vi "XY Graph Get Plot(s) from Headerless String Array.vi"(4 "Default X step (1)":dbl=1.0, 6 "Default X start (0)":dbl, 7 "Alternating Axes?":bool, 8 "error in (no error)":errorcluster, 9 "Delimiter":string, 10 "Abscissa Column? (T)":bool=TRUE, 11 "Text Lines":string[](array[string])) -> (0 "error out":errorcluster, 3 "Plot Array":cluster{"Array":dbl[], "Array":dbl[]}[](array[cluster]))   [LabVIEW 2021, in "XY Graph Add-Ons.lvlib"]
uses:
  XY Graph Add-Ons.lvlib
  1475674b-5358-4f42-8095-6f5b9cc962ed.vi
  95ffc780-ba50-4d26-8739-638f745671cb.vi
  <vilib>/Utility/error.llb/Error Cluster From Error Code.vi
  <vilib>/ErrorRing/Error Ring.xnode
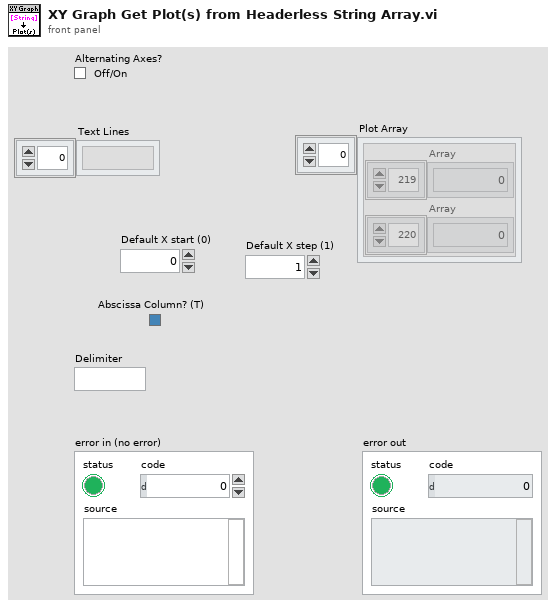
[diagram p1: front panel]
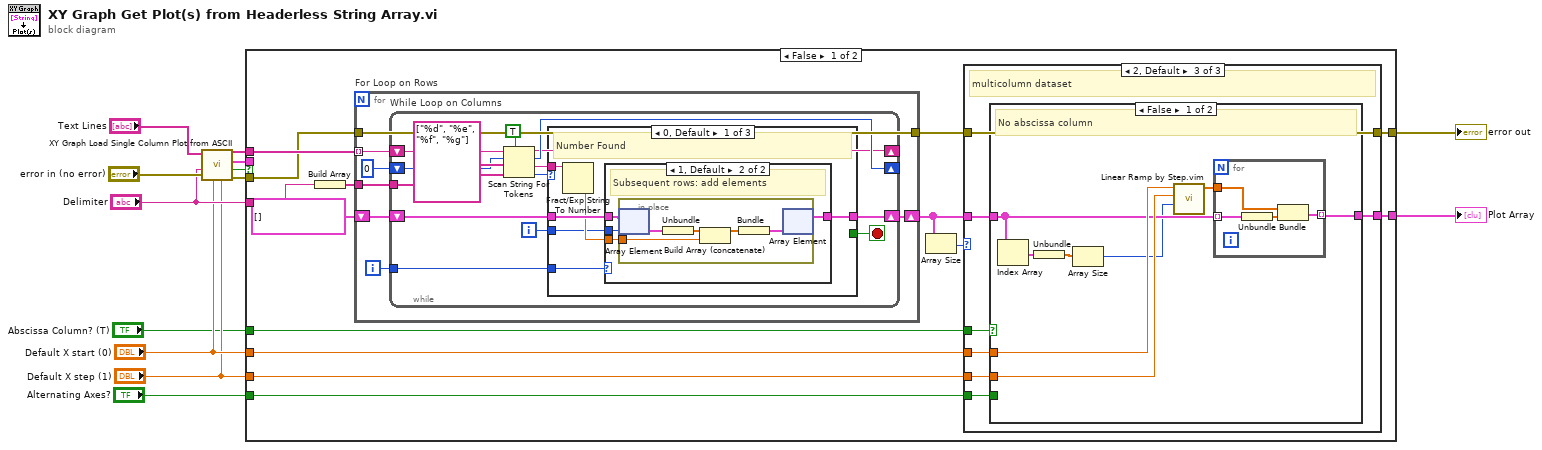
[diagram p0: block diagram]
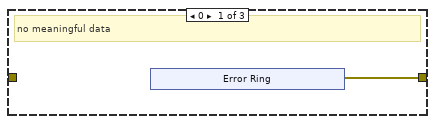
[diagram p2: hidden frame]
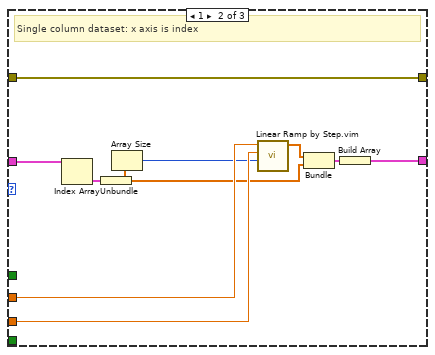
[diagram p3: hidden frame]
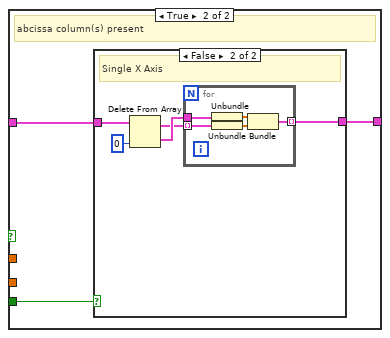
[diagram p4: hidden frame]
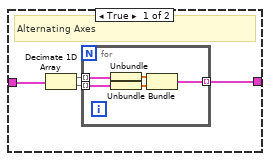
[diagram p5: hidden frame]
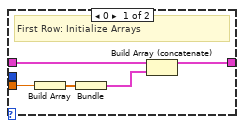
[diagram p6: hidden frame]
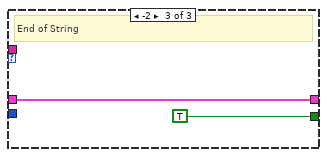
[diagram p8: hidden frame]
diagram:
  n1 = call "XY Graph Load Single Column Plot from ASCII.vi"("Default X step (1)"="Default X step (1)", "Default X start (0)"="Default X start (0)", "error in (no error)"="error in (no error)", "Delimiter (TAB)"="Delimiter", "String Array"="Text Lines") -> ("error out"=w8:errorcluster, "Single Column?"=w9:bool, "Plot Array"=w10:cluster{"Array":dbl[], "Array":dbl[]}[], "String Array dup"=w13:string[])  [unwired: 3 in]
  n2 = case shown="False" w9 {
    tunnel: [w27 w129] -> w4
    tunnel: "Alternating Axes?" -> [w26 _]
    tunnel: [w25 w128] -> w6
    tunnel: w13 -> [w19 _]
    tunnel: "Delimiter" -> [w18 _]
    tunnel: w8 -> [w17 w128]
    tunnel: w10 -> [_ w129]
    tunnel: "Default X start (0)" -> [w16 _]
    tunnel: "Default X step (1)" -> [w15 _]
    tunnel: "Abscissa Column? (T)" -> [w14 _]
    frame False {
      n3 = Build Array(w18) -> (w24:string[])
      n4 = for "For Loop on Rows" {
        tunnel: w19 -> [w90] mode=indexing
        tunnel: w24 -> [w89]
        shift-right: [w86] -> w22
        shift-left: cluster{dbl[]}[] [] -> [w87]
        tunnel: w17 -> [w84]
        tunnel: [w84] -> w20
        i -> [w85]
        n5 = while "While Loop on Columns" {
          tunnel: w89 -> [w103]
          shift-right: [w99] -> _
          shift-left: w90 -> [w104]
          shift-right: [w100] -> _
          shift-left: 0 ("offset past token") -> [w101]
          shift-right: [w93] -> w86
          shift-left: w87 -> [w95]
          tunnel: w85 -> [w92]
          i -> [w94]
          stop <- w96 stop-if-true
          n6 = Scan String For Tokens(5:TRUE ("allow empty tokens? (F)"), 6:w103, 7:string[] ["%d", "%e", "%f", "%g"] ("operators (none)"), 8:w101, 9:w104) -> (0:w98:i32, 1:w97:string, 2:w100:i32, 3:w99:string)  [unwired: 1 in]
          n7 = case shown="0, Default" w98 {
            tunnel: w97 -> [w110 _ _]
            tunnel: [_ _ TRUE] -> w96
            tunnel: w95 -> [w109 w125 w126]
            tunnel: w94 -> [w106 _ _]
            tunnel: [w107 w125 w126] -> w93
            tunnel: w92 -> [w105 _ _]
            frame 0, Default {
              # "Number Found"
              n8 = Fract/Exp String To Number(string=w110) -> (number=w108:dbl)  [unwired: 3 in, 1 out]
              n9 = case shown="1, Default" w105 {
                tunnel: w109 -> [w113 w119]
                tunnel: w108 -> [w115 w118]
                tunnel: [w111 w117] -> w107
                tunnel: w106 -> [_ w116]
                frame 0 {
                  # "First Row: Initialize Arrays"
                  n10 = Build Array(w115) -> (w114:dbl[])
                  n11 = Bundle(w114) -> (w112:cluster{dbl[]})  [unwired: 1 in]
                  n12 = Build Array (concatenate)(w113, w112) -> (w111:cluster{dbl[]}[])
                }
                frame 1, Default {
                  # "Subsequent rows: add elements"
                  n13 = in-place {
                    in-place-border: w118 -> [w123]
                    n14 = in-place-array #1(w119, w116) -> (w124:cluster{dbl[]})
                    n15 = Unbundle(w124) -> (w121:dbl[])
                    n16 = Build Array (concatenate)(w121, w123) -> (w122:dbl[])
                    n17 = Bundle(w122) -> (w120:cluster{dbl[]})  [unwired: 1 in]
                    n18 = in-place-array #1(w120) -> (w117:cluster{dbl[]}[])  [unwired: 1 out]
                  }
                }
              }
            }
            frame -1 {
              # "Some columns have less numbers than others"
              # "Number not Found"
            }
            frame -2 {
              # "End of String"
            }
          }
        }
      }
      n19 = Array Size(array=w22) -> (size(s)=w21:i32)
      n20 = case shown="2, Default" w21 {
        tunnel: [_ w39 w49] -> w27
        tunnel: w26 -> [_ _ w48]
        tunnel: w22 -> [_ w42 w47]
        tunnel: w20 -> [_ w38 w46]
        tunnel: [w28 w38 w46] -> w25
        tunnel: w16 -> [_ w37 w44]
        tunnel: w15 -> [_ w36 w43]
        tunnel: w14 -> [_ _ w45]
        frame 0 {
          # "no meaningful data"
          n21 = xnode "Error Ring"() -> ("error out"=w28:errorcluster)
        }
        frame 1 {
          # "Single column dataset: x axis is index"
          n22 = Index Array(array=w42) -> (element=w41:cluster{dbl[]})  [unwired: 1 in]
          n23 = Unbundle(w41) -> (w35:dbl[])
          n24 = Array Size(array=w35) -> (size(s)=w34:i32)
          n25 = call "Linear Ramp by Step.vim"("# Elements (1)"=w34, "Step (1)"=w36, "Start (0)"=w37) -> ("Ramp"=w33:dbl[])  [unwired: 8 in]
          n26 = Bundle("Ramp"=w33, w35) -> (w40:cluster{"Ramp":dbl[], dbl[]})  [unwired: 1 in]
          n27 = Build Array(w40) -> (w39:cluster{"Ramp":dbl[], dbl[]}[])
        }
        frame 2, Default {
          # "multicolumn dataset"
          n28 = case shown="False" w45 {
            tunnel: [w50 w64] -> w49
            tunnel: w48 -> [_ w63]
            tunnel: w47 -> [w55 w62]
            tunnel: w44 -> [w57 _]
            tunnel: w43 -> [w56 _]
            frame False {
              # "No abscissa column"
              n29 = Index Array(array=w55) -> (element=w54:cluster{dbl[]})  [unwired: 1 in]
              n30 = Unbundle(w54) -> (w53:dbl[])
              n31 = Array Size(array=w53) -> (size(s)=w52:i32)
              n32 = call "Linear Ramp by Step.vim"("# Elements (1)"=w52, "Step (1)"=w56, "Start (0)"=w57) -> ("Ramp"=w51:dbl[])  [unwired: 8 in]
              n33 = for {
                tunnel: w55 -> [w61] mode=indexing
                tunnel: [w59] -> w50 mode=indexing
                tunnel: w51 -> [w58]
                n34 = Unbundle(w61) -> (w60:dbl[])
                n35 = Bundle("Ramp"=w58, w60) -> (w59:cluster{"Ramp":dbl[], dbl[]})  [unwired: 1 in]
              }
            }
            frame True {
              # "abcissa column(s) present"
              n36 = case shown="False" w63 {
                tunnel: w62 -> [w68 w77]
                tunnel: [w65 w78] -> w64
                frame True {
                  # "Alternating Axes"
                  n37 = Decimate 1D Array(w68) -> (w67:cluster{dbl[]}[], w66:cluster{dbl[]}[])
                  n38 = for {
                    tunnel: w67 -> [w73] mode=indexing
                    tunnel: w66 -> [w72] mode=indexing
                    tunnel: [w69] -> w65 mode=indexing
                    n39 = Unbundle(w73) -> (w71:dbl[])
                    n40 = Unbundle(w72) -> (w70:dbl[])
                    n41 = Bundle(w71, w70) -> (w69:cluster{dbl[], dbl[]})  [unwired: 1 in]
                  }
                }
                frame False {
                  # "Single X Axis"
                  n42 = Delete From Array(array=w77, index=0) -> (deleted portion=w75:cluster{dbl[]}, array with subset deleted=w74:cluster{dbl[]}[])  [unwired: 1 in]
                  n43 = for {
                    tunnel: w75 -> [w83]
                    tunnel: w74 -> [w82] mode=indexing
                    tunnel: [w79] -> w78 mode=indexing
                    n44 = Unbundle(w83) -> (w81:dbl[])
                    n45 = Unbundle(w82) -> (w80:dbl[])
                    n46 = Bundle(w81, w80) -> (w79:cluster{dbl[], dbl[]})  [unwired: 1 in]
                  }
                }
              }
            }
          }
        }
      }
    }
    frame True {
    }
  }
  "error out" <- w6
  "Plot Array" <- w4
